vi "Facade.vi"(0 "Data In":T4, 2 "Display State In":T2={"MaxPage"=10}, 3 "Container State":T3) -> (6 "Data Out":T4, 7 "Display State Out":T2={"MaxPage"=10}, 8 "Action":T1)   [LabVIEW 2017, in "Page-XControl.xctl"]
uses:
  Page-XControl.xctl
  Data.ctl
  <vilib>/_xctls/Container State.ctl
  State.ctl
  <vilib>/_xctls/Action.ctl
  <vilib>/_xctls/XControlSupport.lvlib
panel:
  in  "PageNumber":u32 caption="Numeric"
  out "PageString":string caption="String"
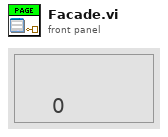
[diagram p1: front panel]
types:
  T1 = typedef "XControlSupport.lvlib/Action.ctl" = cluster{"Data Changed?":bool, "State Changed?":bool, "Action Name":string}
  T2 = typedef "Page-XControl.xctl/State.ctl" = cluster{"MaxPage":u32}
  T3 = typedef "XControlSupport.lvlib/Container State.ctl" = cluster{"Indicator?":bool, "Run Mode?":bool, " Refnum":refnum<vi>}
  T4 = typedef "Page-XControl.xctl/Data.ctl" = u32
  T5 = enum8{"Enabled", "Disabled", "Disabled and Grayed Out"}
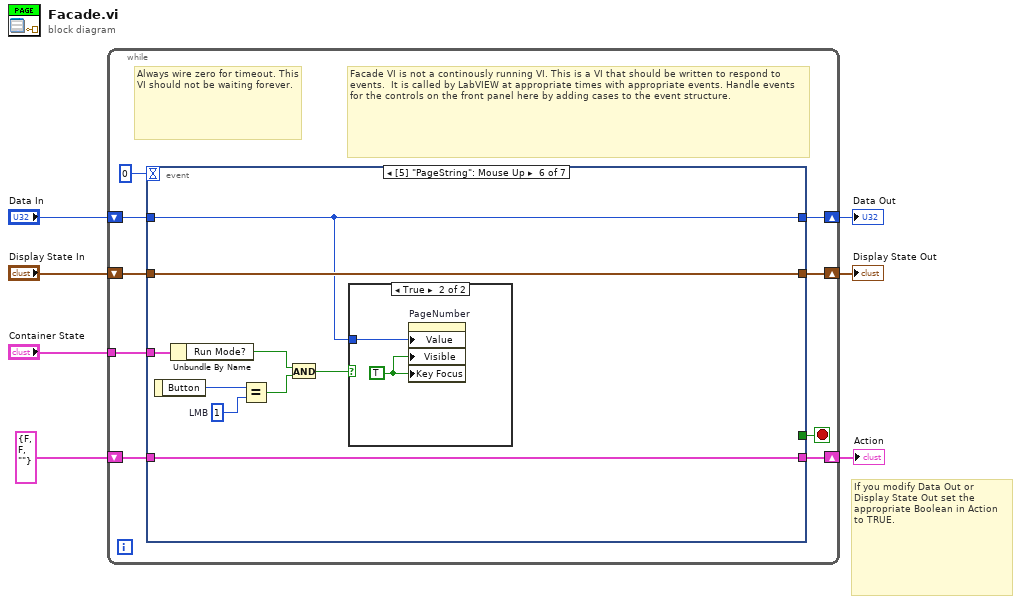
[diagram p0: block diagram]
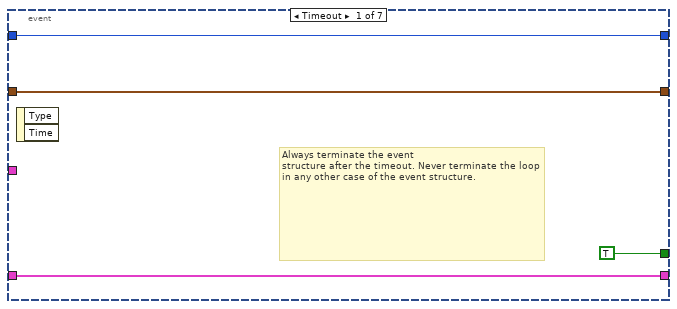
[diagram p2: hidden frame]
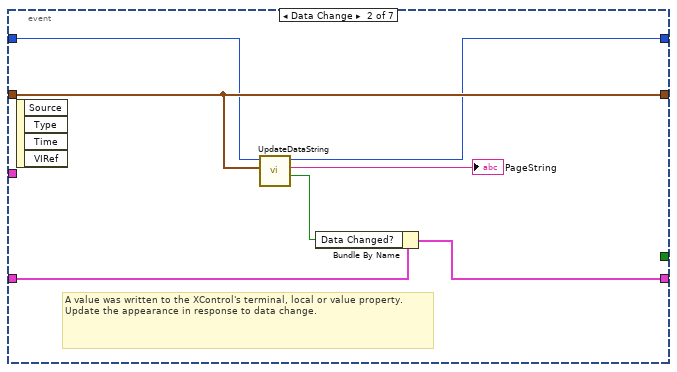
[diagram p3: hidden frame]
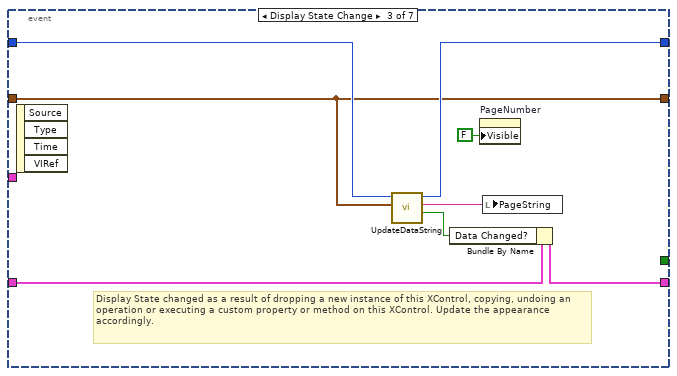
[diagram p4: hidden frame]
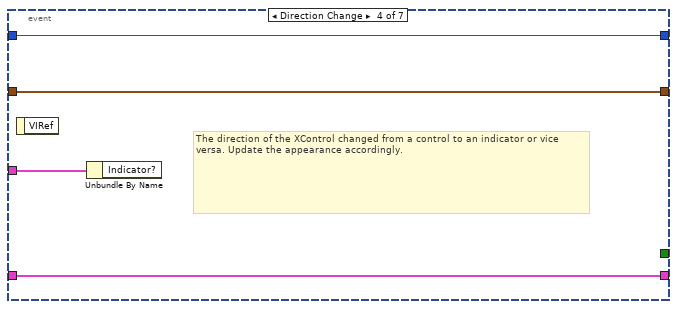
[diagram p5: hidden frame]
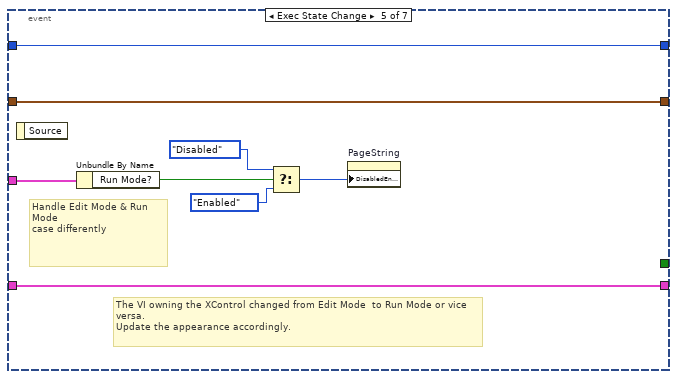
[diagram p6: hidden frame]
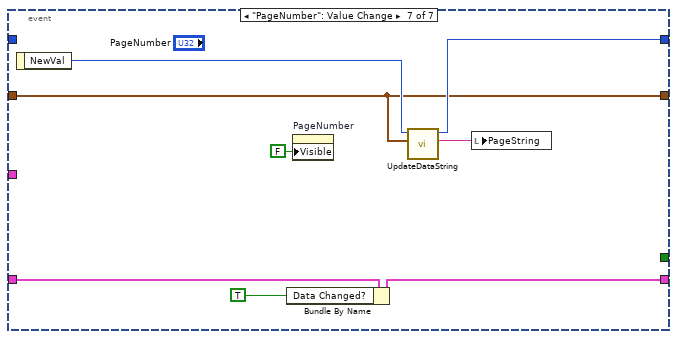
[diagram p8: hidden frame]
diagram:
  # "If you modify Data Out or\nDisplay State Out set the\nappropriate Boolean in Action\nto TRUE."
  n1 = while {
    shift-right: [w16] -> w4
    shift-left: "Display State In" -> [w8]
    tunnel: "Container State" -> [w13]
    shift-right: [w11] -> w7
    shift-left: "Data In" -> [w12]
    shift-right: [w9] -> w2
    shift-left: T1 {"Data Changed?"=FALSE, "State Changed?"=FALSE, "Action Name"=""} ("Action") -> [w10]
    stop <- w15 stop-if-true
    # "Facade VI is not a continously running VI. This is a VI that should be written to respond to events.  It is called by LabVIEW at appropriate times with appropriate events. Handle events for the controls on the front panel here by adding cases to the event structure."
    # "Always wire zero for timeout. This\nVI should not be waiting forever."
    n2 = event shown="[5] \"PageString\": Mouse Up" {
      selector: _ -> [_ _ _ _ _ _ _]
      dyn-events: _ -> [_ _ _ _ _ _ _]
      timeout: 0 -> [_ _ _ _ _ _ _]
      tunnel: w8 -> [w18 w26 w28 w38 w46 w56 w59]
      tunnel: [w18 w26 w28 w38 w46 w56 w59] -> w16
      tunnel: [TRUE _ _ _ _ _ _] -> w15
      tunnel: w13 -> [_ _ _ w39 w47 w51 _]
      tunnel: w12 -> [w17 w24 w32 w37 w45 w52 _]
      tunnel: [w17 w23 w29 w37 w45 w52 w60] -> w11
      tunnel: [w19 w22 w31 w36 w44 w55 w65] -> w9
      tunnel: w10 -> [w19 w27 w35 w36 w44 w55 w66]
      event Timeout {
        # "Always terminate the event\nstructure after the timeout. Never terminate the loop in any other case of the event structure."
        n3 = event-data() -> ()  [unwired: 1 in, 2 out]
      }
      event Data Change {
        # "A value was written to the XControl's terminal, local or value property.\nUpdate the appearance in response to data change."
        n4 = event-data() -> ()  [unwired: 1 in, 4 out]
        n5 = call "UpdateDataString.vi"("Display State In"=w26, "Data In"=w24) -> ("Data Changed?"=w21:bool, "Display String"=→"PageString":string, "lower limit"=w23:T4)  [unwired: 7 in]
        n6 = Bundle By Name(cluster=w27, "Data Changed?"=w21) -> (w22:T1)
      }
      event Display State Change {
        # "Display State changed as a result of dropping a new instance of this XControl, copying, undoing an operation or executing a custom property or method on this XControl. Update the appearance accordingly."
        n7 = event-data() -> ()  [unwired: 1 in, 4 out]
        n8 = call "UpdateDataString.vi"("Display State In"=w28, "Data In"=w32) -> ("Data Changed?"=w30:bool, "Display String"=w33:string, "lower limit"=w29:T4)  [unwired: 7 in]
        n9 = Bundle By Name(cluster=w35, "Data Changed?"=w30) -> (w31:T1)
        n10 = property on="PageNumber" class="DigNum (strict)"("Visible"=FALSE) -> ()  [unwired: 2 in, 2 out]
        n11 = local write "PageString"(w33) -> ()
      }
      event Direction Change {
        # "The direction of the XControl changed from a control to an indicator or vice versa. Update the appearance accordingly."
        n12 = event-data() -> ()  [unwired: 1 in, 1 out]
        n13 = Unbundle By Name(w39) -> ()  [unwired: 1 out]
      }
      event Exec State Change {
        # "The VI owning the XControl changed from Edit Mode  to Run Mode or vice versa.\nUpdate the appearance accordingly."
        # "Handle Edit Mode & Run Mode\ncase differently"
        n14 = event-data() -> ()  [unwired: 1 in, 1 out]
        n15 = Unbundle By Name(w47) -> ("Run Mode?"=w43:bool)
        n16 = Select(t=T5."Disabled" ("Disabled"), s=w43, f=T5."Enabled" ("Disabled")) -> (s? t:f=w40:T5)
        n17 = property on="PageString" class="Str"("DisabledEnum"=w40) -> ()  [unwired: 2 in, 2 out]
      }
      event "PageString": Mouse Up {
        w53 = u16 1  # LMB
        n18 = event-data() -> ("Button"=w54:u16)  [unwired: 1 in]
        n19 = Unbundle By Name(w51) -> ("Run Mode?"=w49:bool)
        n20 = Equal?(x=w54, y=w53) -> (x = y?=w50:bool)
        n21 = And(x=w49, y=w50) -> (x .and. y?=w48:bool)
        n22 = case shown="True" w48 {
          tunnel: w52 -> [_ w57]
          frame False {
          }
          frame True {
            w58 = TRUE
            n23 = property on="PageNumber" class="DigNum (strict)"("Value"=w57, "Visible"=w58, "Key Focus"=w58) -> ()  [unwired: 2 in, 2 out]
          }
        }
      }
      event "PageNumber": Value Change {
        n24 = event-data() -> ("NewVal"=w61:u32)  [unwired: 1 in]
        n25 = Bundle By Name(cluster=w66, "Data Changed?"=TRUE) -> (w65:T1)
        n26 = property on="PageNumber" class="DigNum (strict)"("Visible"=FALSE) -> ()  [unwired: 2 in, 2 out]
        n27 = call "UpdateDataString.vi"("Display State In"=w59, "Data In"=w61) -> ("Display String"=w62:string, "lower limit"=w60:T4)  [unwired: 7 in, 1 out]
        n28 = local write "PageString"(w62) -> ()
      }
    }
  }
  "Display State Out" <- w4
  "Data Out" <- w7
  "Action" <- w2
